vi "GetPcName.vi"(8 "error in (no error)":errorcluster) -> (0 "error out":errorcluster, 1 "IP":string, 2 "Basic Name":string, 3 "Computer Full Name":string)   [LabVIEW 2013]
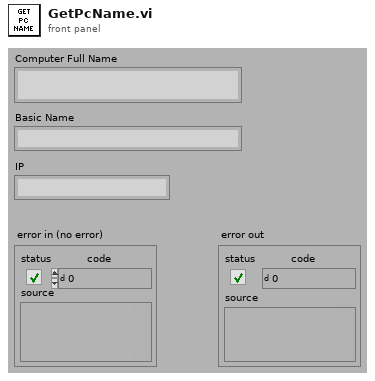
[diagram p1: front panel]
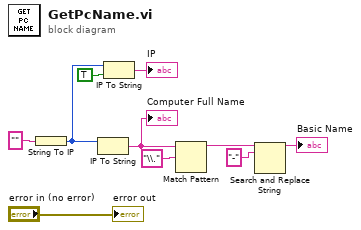
[diagram p0: block diagram]
diagram:
  n1 = String To IP(1:"" ("name")) -> (0:w7:u32)
  n2 = IP To String(2:w7) -> (0:w9:string)  [unwired: 1 in]
  "Computer Full Name" <- w9
  n3 = IP To String(1:TRUE ("dot notation? (F)"), 2:w7) -> (0:→"IP":string)
  n4 = Match Pattern(string=w9, regular expression="\\.") -> (before substring=w3:string)  [unwired: 1 in, 3 out]
  n5 = Search and Replace String(input string=w3, search string="-") -> (result string=→"Basic Name":string)  [unwired: 6 in, 3 out]
  "error out" <- "error in (no error)"
